vi "Enter Pre-Operational.vi"(8 "error in":errorcluster, 10 "Node-ID":u8, 11 "ICommunicate":refnum<class "ICommunicate.lvclass">) -> (0 "error out":errorcluster)   [LabVIEW 2024, in "Network Mangement.lvclass"]
uses:
  Network Mangement.lvclass
  HAL/Source/Interfaces/ICommunicate/ICommunicate.lvclass
  source/CANopen Message/CANopen Message.lvclass
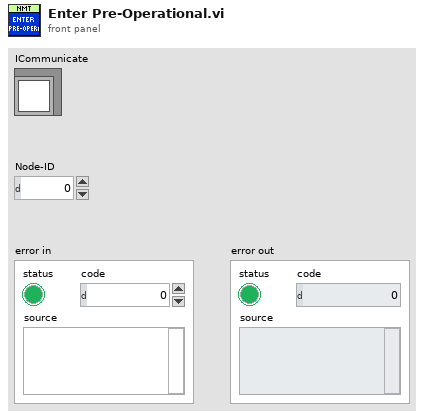
[diagram p1: front panel]
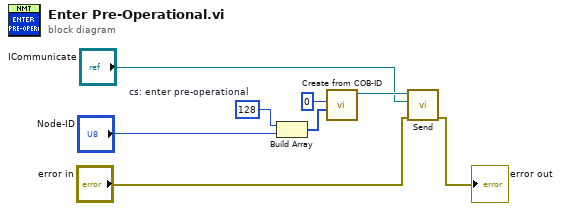
[diagram p0: block diagram]
diagram:
  w6 = u8 128  # cs: enter pre-operational
  n1 = Build Array(w6, "Node-ID") -> (w5:u8[])
  n2 = call "Create from COB-ID.vi"("Data"=w5, "COB-ID"=u32 0) -> ("CANopen Message out"=w7:refnum<class "CANopen Message.lvclass">)  [unwired: 9 in]
  n3 = call "Send.vi"("error in"="error in", "ICommunicate"="ICommunicate", "CANopen Message in"=w7) -> ("error out"=→"error out":errorcluster)  [unwired: 7 in, 1 out]
